vi "Trans Area Check Case.vi"(11 "ResultIn":variant[](array[variant])) -> (3 "Case":i32)   [LabVIEW 2019]
uses:
  Controls/Area Check/Area Check_Result.ctl
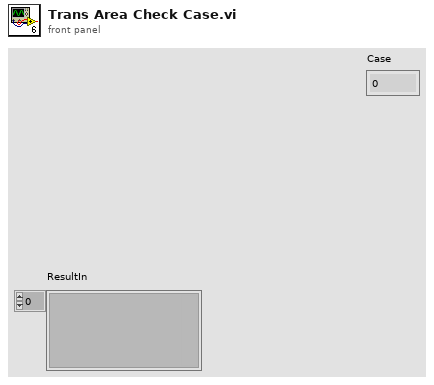
[diagram p1: front panel]
types:
  T1 = typedef "Area Check_Result.ctl" = cluster{"AreaDataOut":cluster{"AreaDataOut":cluster{"Rectangle":T2, "Particle Measurements (Pixels)":dbl[][]}}[], "Percent":dbl[], "Item?":bool, "ROI":i32[]}
  T2 = typedef "IMAQ Rectangle" = cluster{"Left":i32, "Top":i32, "Right":i32, "Bottom":i32, "Rotation":dbl}
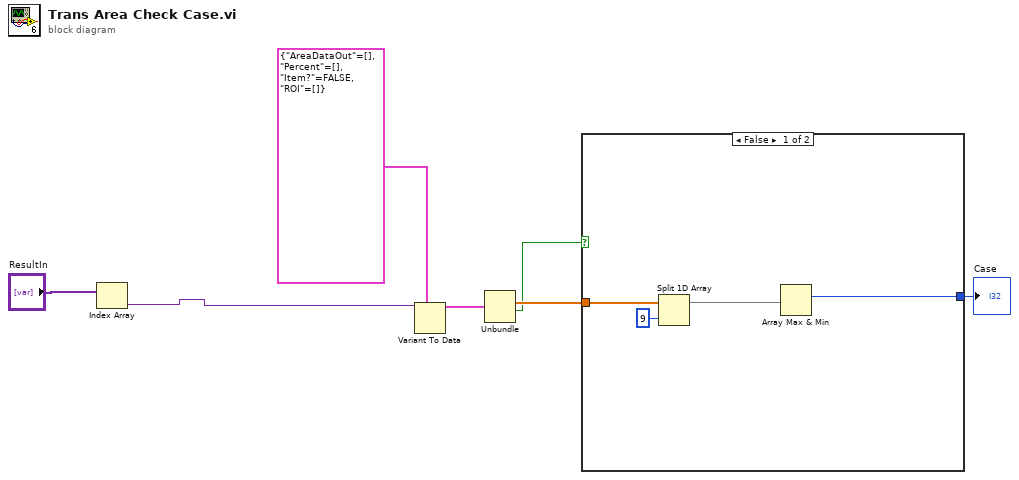
[diagram p0: block diagram]
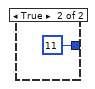
[diagram p2: hidden frame]
diagram:
  n1 = Index Array(array="ResultIn") -> (element=w1:variant)  [unwired: 1 in]
  n2 = Variant To Data(type=T1 {"AreaDataOut"=[], "Percent"=[], "Item?"=FALSE, "ROI"=[]} ("cluster"), Variant=w1) -> (data=w6:T1)  [unwired: 1 in, 1 out]
  n3 = Unbundle(w6) -> ("Percent"=w5:dbl[], "Item?"=w4:bool)  [unwired: 2 out]
  n4 = case shown="False" w4 {
    tunnel: w5 -> [w10 _]
    tunnel: [w11 11] -> w3
    frame False {
      n5 = Split 1D Array(array=w10, index=9) -> (first subarray=w8:dbl[])  [unwired: 1 out]
      n6 = Array Max & Min(array=w8) -> (max index (indices)=w11:i32)  [unwired: 3 out]
    }
    frame True {
    }
  }
  "Case" <- w3
